vi "Band Phase (Orders).vi"(0 "Cross phase [degrees]":cluster{"f0":dbl, "df":dbl, "phase":sgl[]}, 1 "Speed (RPM)":sgl, 5 "Start":dbl, 7 "Stop":dbl, 11 "error in (no error)":errorcluster) -> (6 "Phase (deg)":sgl, 15 "error out":errorcluster)   [LabVIEW 2017, in "VibrationAnalysisFunctions.lvlib"]
uses:
  <vilib>/addons/InsightCM/Utilities/Analysis/Vibration/VibrationAnalysisFunctions.lvlib
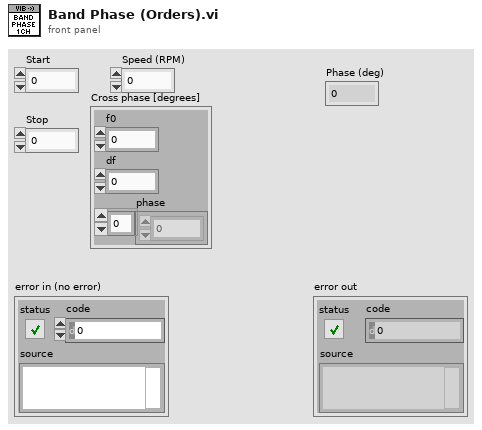
[diagram p1: front panel]
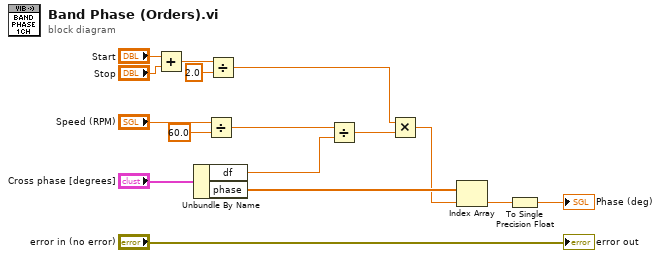
[diagram p0: block diagram]
diagram:
  n1 = Add(x="Start", y="Stop") -> (x+y=w3:dbl)
  n2 = Unbundle By Name("Cross phase [degrees]") -> ("df"=w8:dbl, "phase"=w11:sgl[])
  n3 = Divide(x="Speed (RPM)", y=60.0) -> (x/y=w9:dbl)
  n4 = Divide(x=w3, y=2.0) -> (x/y=w1:dbl)
  n5 = Divide(x=w9, y=w8) -> (x/y=w7:dbl)
  n6 = Multiply(x=w1, y=w7) -> (x*y=w6:dbl)
  n7 = Index Array(array=w11, index=w6) -> (element=w10:sgl)
  n8 = To Single Precision Float(number=w10) -> (single precision float=→"Phase (deg)":sgl)
  "error out" <- "error in (no error)"
